vi "Graph Example.vi"() -> ()   [LabVIEW 2016, in "PanelExample.lvclass"]
uses:
  PanelExample.lvclass
  PanelObject/PanelObject.lvclass
  PanelDataNode/PanelDataNode.lvclass
  PanelDataNode/PanelDataNode.lvclass/PanelDataNode.ctl
  PanelDataNode/Split Mode.ctl
  <vilib>/Analysis/baseanly.llb/Mean (DBL).vi
  <vilib>/measure/NI_MABase.lvlib
  <vilib>/Analysis/NI_AALBase.lvlib
  QueueManager.llb/Insert.vi
panel:
  in  "Node*":refnum<data-value>
  out "波形图表":waveform(dbl)(graph)={"t0"=timestamp(9406.0 s since 1904-01-01), "dt"=0.001, "Y"=array[1000 elements]}
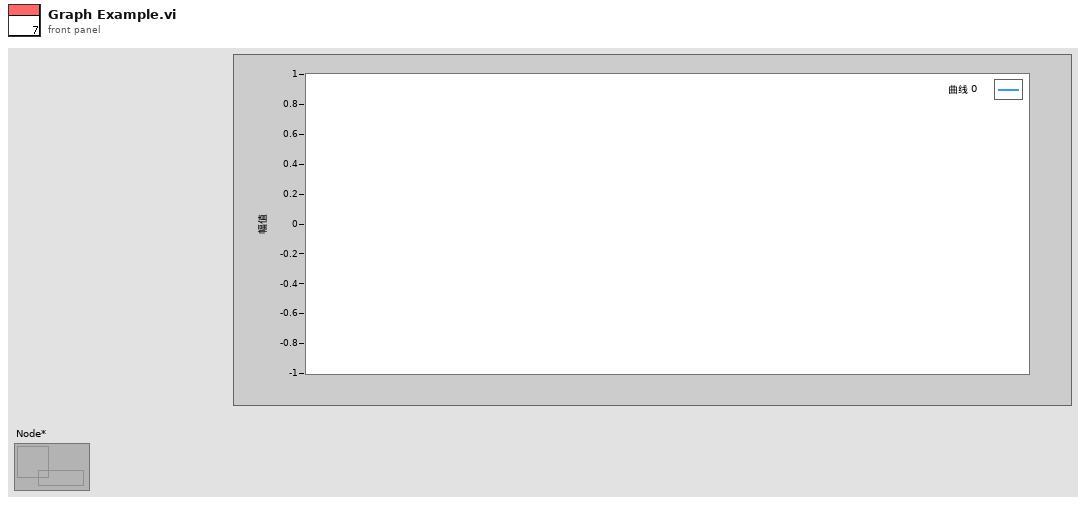
[diagram p1: front panel]
types:
  T1 = enum16{"Sine Wave", "Triangle Wave", "Square Wave", "Sawtooth Wave"}
  T2 = typedef "PanelDataNode.lvclass/Split Mode.ctl" = enum16{"Horizontal(up)", "Vertical(left)", "Horizontal(down)", "Vertical(right)"}
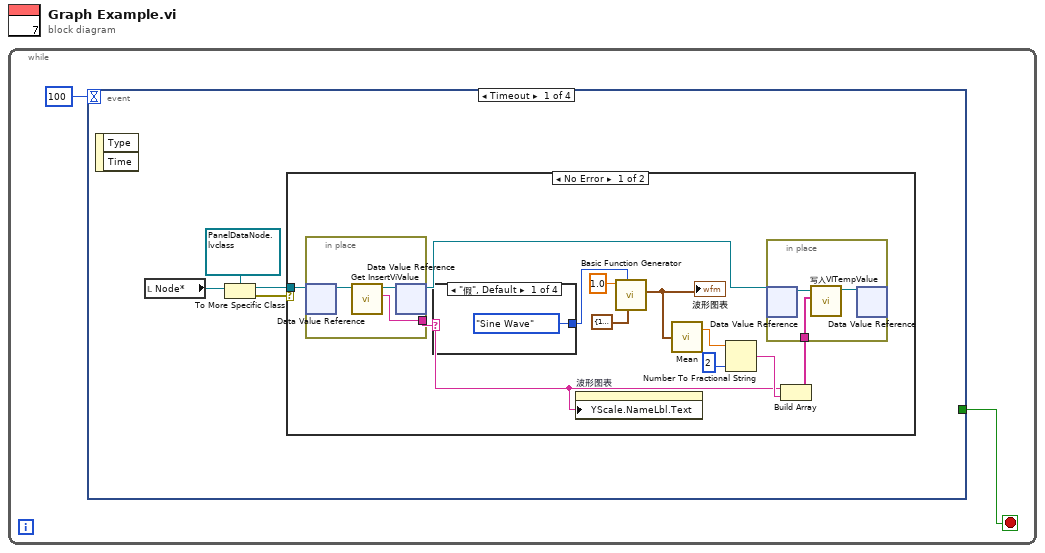
[diagram p0: block diagram]
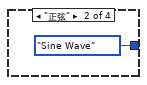
[diagram p2: hidden frame]
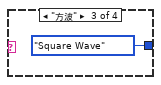
[diagram p3: hidden frame]
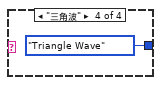
[diagram p4: hidden frame]
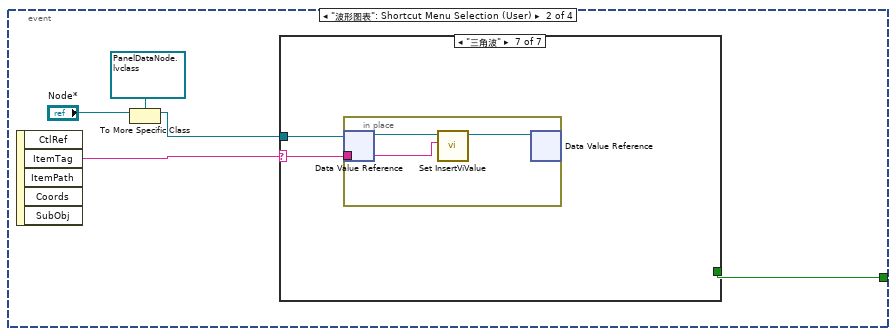
[diagram p6: hidden frame]
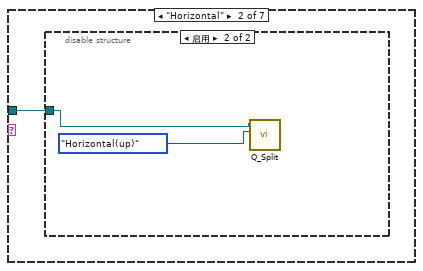
[diagram p8: hidden frame]
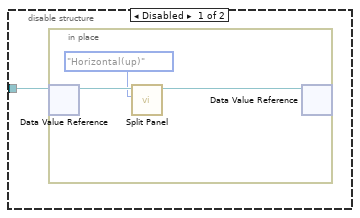
[diagram p9: hidden frame]
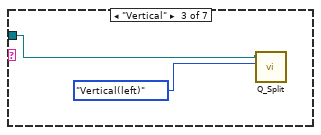
[diagram p10: hidden frame]
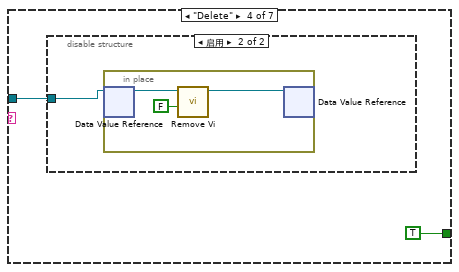
[diagram p11: hidden frame]
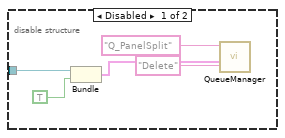
[diagram p12: hidden frame]
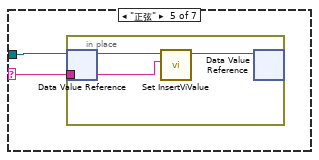
[diagram p13: hidden frame]
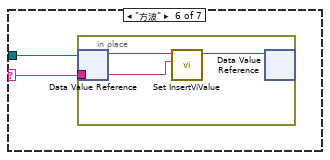
[diagram p14: hidden frame]
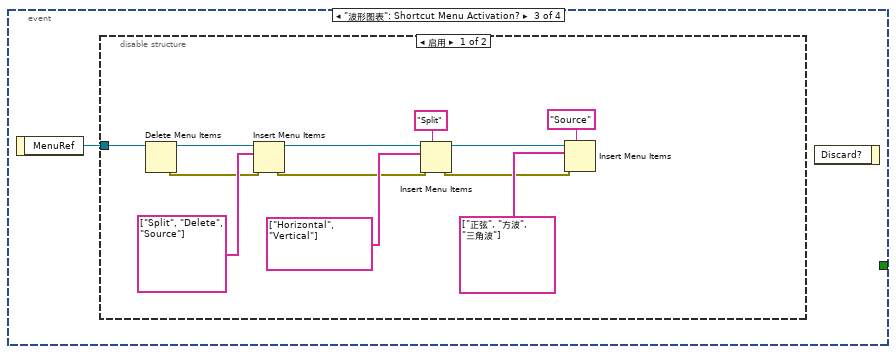
[diagram p15: hidden frame]
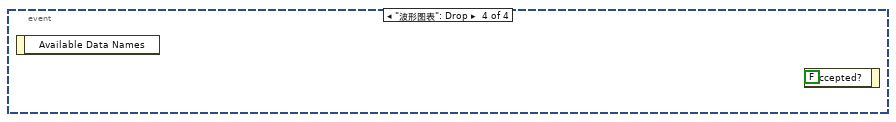
[diagram p17: hidden frame]
diagram:
  n1 = while {
    stop <- w1 stop-if-true
    n2 = event shown="[0] Timeout" {
      selector: _ -> [_ _ _ _]
      dyn-events: _ -> [_ _ _ _]
      timeout: 100 -> [_ _ _ _]
      tunnel: [_ w28 _ _] -> w1
      event Timeout {
        n3 = event-data() -> ()  [unwired: 1 in, 2 out]
        n4 = local read "Node*"() -> (w5:refnum<data-value>)
        n5 = To More Specific Class(target class=refnum<data-value> refnum ("Node*"), reference=w5) -> (specific class reference=w3:refnum<data-value>, error out=w4:errorcluster)  [unwired: 1 in]
        n6 = case shown="No Error" w4 {
          tunnel: w3 -> [w15 _]
          frame No Error {
            n7 = in-place {
              in-place-border: [w25] -> w7
              n8 = in-place-dvr #1(w15) -> (w27:refnum<class "PanelDataNode.lvclass">)  [unwired: 1 out]
              n9 = call-dynamic "Get InsertViValue.vi"("PanelDataNode 输入"=w27) -> ("ViValue"=w25:string, "PanelDataNode 输出"=w26:refnum<class "PanelDataNode.lvclass">)  [unwired: 8 in, 1 out]
              n10 = in-place-dvr #1(w26) -> (w12:refnum<data-value>)  [unwired: 1 out]
            }
            n11 = case shown="\"假\", Default" w7 {
              tunnel: [T1."Sine Wave" ("signal type") T1."Sine Wave" ("signal type") T1."Square Wave" ("signal type") T1."Triangle Wave" ("signal type")] -> w14
              frame "假", Default {
              }
              frame "正弦" {
              }
              frame "方波" {
              }
              frame "三角波" {
              }
            }
            n12 = property on="波形图表" class="WFChart (strict)"("YScale.NameLbl.Text"=w7) -> ()  [unwired: 2 in, 2 out]
            n13 = call <vilib>:"Basic Function Generator.vi"("sampling info"=cluster{"Fs":dbl, "#s":dbl} {"Fs"=100.0, "#s"=101.0}, "signal type"=w14, "frequency"=1.0) -> ("signal out"=w13:waveform(dbl))  [unwired: 6 in, 2 out]
            "波形图表" <- w13
            n14 = call-poly <vilib>:"Mean.vi"("X"=w13) -> ("mean"=w11:dbl)  [unwired: 1 out]
            n15 = Number To Fractional String(number=w11, precision (6)=i16 2 ("精度(6)")) -> (F-format string=w9:string)  [unwired: 2 in]
            n16 = Build Array(w7, w9) -> (w8:string[])
            n17 = in-place {
              in-place-border: w8 -> [w18]
              n18 = in-place-dvr #2(w12) -> (w20:refnum<class "PanelDataNode.lvclass">)  [unwired: 1 out]
              n19 = call "写入VITempValue.vi"("VITempValue"=w18, "PanelDataNode输入"=w20) -> ("PanelDataNode输出"=w19:refnum<class "PanelDataNode.lvclass">)  [unwired: 8 in, 1 out]
              n20 = in-place-dvr #2(w19) -> ()  [unwired: 2 out]
            }
          }
          frame Error {
          }
        }
      }
      event "波形图表": Shortcut Menu Selection (User) {
        n21 = event-data() -> ("ItemTag"=w32:string)  [unwired: 1 in, 4 out]
        n22 = To More Specific Class(target class=refnum<data-value> refnum ("Node*"), reference="Node*") -> (specific class reference=w29:refnum<data-value>)  [unwired: 1 in, 1 out]
        n23 = case shown="\"三角波\"" w32 {
          selector: w32 -> [_ _ _ _ w53 w58 w63]
          tunnel: w29 -> [_ w33 w41 w42 w54 w59 w64]
          tunnel: [_ _ _ TRUE _ _ _] -> w28
          frame "假", Default {
          }
          frame "Horizontal" {
            n24 = disable-structure shown="启用" {
              disable-tunnel: w33 -> [w34 w39]
              frame Disabled {
                n25 = in-place {
                  n26 = in-place-dvr #3(w34) -> (w37:refnum<class "PanelDataNode.lvclass">)  [unwired: 1 out]
                  n27 = call-dynamic "Split Panel.vi"("Split Mode"=Split_Mode."Horizontal(up)", "PanelDataNode 输入"=w37) -> ("PanelDataNode 输出"=w36:refnum<class "PanelDataNode.lvclass">)  [unwired: 7 in, 2 out]
                  n28 = in-place-dvr #3(w36) -> ()  [unwired: 2 out]
                }
              }
              frame Enabled {
                n29 = call "Q_Split.vi"("Split Mode"=Split_Mode."Horizontal(up)", "ChildNode*"=w39) -> ()  [unwired: 9 in, 1 out]
              }
            }
          }
          frame "Vertical" {
            n30 = call "Q_Split.vi"("Split Mode"=Split_Mode."Vertical(left)", "ChildNode*"=w41) -> ()  [unwired: 9 in, 1 out]
          }
          frame "Delete" {
            n31 = disable-structure shown="启用" {
              disable-tunnel: w42 -> [w48 w49]
              frame Disabled {
                n32 = Bundle("Node*"=w48, TRUE) -> (w46:cluster{"Node*":refnum<data-value>, bool})  [unwired: 1 in]
                n33 = call-poly "QueueManager.vi"("Data"=w46, "Event"="Delete", "QueueName"="Q_PanelSplit") -> ()  [unwired: 7 in, 2 out]
              }
              frame Enabled {
                n34 = in-place {
                  n35 = in-place-dvr #4(w49) -> (w52:refnum<class "PanelDataNode.lvclass">)  [unwired: 1 out]
                  n36 = call-dynamic "Remove Vi.vi"("Abort VI"=FALSE, "PanelDataNode 输入"=w52) -> ("PanelDataNode 输出"=w51:refnum<class "PanelDataNode.lvclass">)  [unwired: 6 in, 3 out]
                  n37 = in-place-dvr #4(w51) -> ()  [unwired: 2 out]
                }
              }
            }
          }
          frame "正弦" {
            n38 = in-place {
              in-place-border: w53 -> [w56]
              n39 = in-place-dvr #5(w54) -> (w57:refnum<class "PanelDataNode.lvclass">)  [unwired: 1 out]
              n40 = call-dynamic "Set InsertViValue.vi"("ViValue"=w56, "PanelDataNode 输入"=w57) -> ("PanelDataNode 输出"=w55:refnum<class "PanelDataNode.lvclass">)  [unwired: 8 in, 1 out]
              n41 = in-place-dvr #5(w55) -> ()  [unwired: 2 out]
            }
          }
          frame "方波" {
            n42 = in-place {
              in-place-border: w58 -> [w61]
              n43 = in-place-dvr #6(w59) -> (w62:refnum<class "PanelDataNode.lvclass">)  [unwired: 1 out]
              n44 = call-dynamic "Set InsertViValue.vi"("ViValue"=w61, "PanelDataNode 输入"=w62) -> ("PanelDataNode 输出"=w60:refnum<class "PanelDataNode.lvclass">)  [unwired: 8 in, 1 out]
              n45 = in-place-dvr #6(w60) -> ()  [unwired: 2 out]
            }
          }
          frame "三角波" {
            n46 = in-place {
              in-place-border: w63 -> [w66]
              n47 = in-place-dvr #7(w64) -> (w67:refnum<class "PanelDataNode.lvclass">)  [unwired: 1 out]
              n48 = call-dynamic "Set InsertViValue.vi"("ViValue"=w66, "PanelDataNode 输入"=w67) -> ("PanelDataNode 输出"=w65:refnum<class "PanelDataNode.lvclass">)  [unwired: 8 in, 1 out]
              n49 = in-place-dvr #7(w65) -> ()  [unwired: 2 out]
            }
          }
        }
      }
      event "波形图表": Shortcut Menu Activation? {
        n50 = event-data() -> ("MenuRef"=w68:refnum<k9>)  [unwired: 1 in]
        n51 = disable-structure shown="启用" {
          disable-tunnel: w68 -> [w80 _]
          frame Enabled {
            n52 = Delete Menu Items(9:w80) -> (0:w71:errorcluster, 3:w79:refnum<k9>)  [unwired: 3 in]
            n53 = Insert Menu Items(6:w71, 8:string[] ["Split", "Delete", "Source"] ("项名称"), 9:w79) -> (0:w70:errorcluster, 3:w77:refnum<k9>)  [unwired: 3 in, 1 out]
            n54 = Insert Menu Items(5:"Split" ("菜单标识符"), 6:w70, 8:string[] ["Horizontal", "Vertical"], 9:w77) -> (0:w69:errorcluster, 3:w74:refnum<k9>)  [unwired: 2 in, 1 out]
            n55 = Insert Menu Items(5:"Source" ("菜单标识符"), 6:w69, 8:string[] ["正弦", "方波", "三角波"] ("项名称"), 9:w74) -> ()  [unwired: 2 in, 3 out]
          }
          frame Disabled {
          }
        }
        n56 = event-data() -> ()  [unwired: 2 in, 1 out]
      }
      event "波形图表": Drop {
        n57 = event-data() -> ()  [unwired: 1 in, 1 out]
        n58 = event-data("Accepted?"=FALSE ("接受？")) -> ()  [unwired: 1 in, 1 out]
      }
    }
  }
